vi "ProstSpecFormat.vi"(1 "Spectra.txt old (string)":string) -> (0 "Spectra.txt new out":string)   [LabVIEW 2022 SP3]
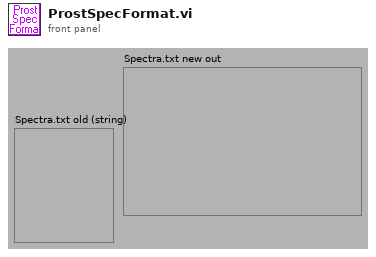
[diagram p1: front panel]
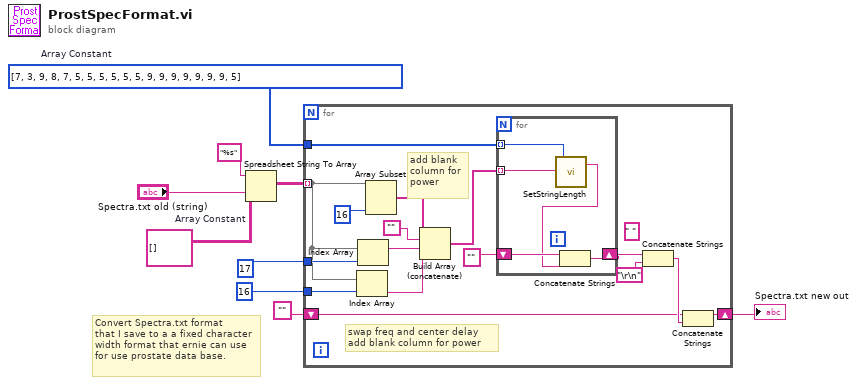
[diagram p0: block diagram]
diagram:
  w6 = i32[] [7, 3, 9, 8, 7, 5, 5, 5, 5, 5, 5, 9, 9, 9, 9, 9, 9, 9, 5]  # Array Constant
  w8 = string[][] []  # Array Constant
  # "Convert Spectra.txt format\nthat I save to a a fixed character\nwidth format that ernie can use\nfor use prostate data base."
  n1 = Spreadsheet String To Array(format string="%s", spreadsheet string="Spectra.txt old (string)", array type (2D Dbl)=w8) -> (array=w7:string[][])  [unwired: 1 out]
  n2 = for {
    tunnel: w7 -> [w10] mode=indexing
    tunnel: w6 -> [w25]
    shift-right: [w23] -> w2
    shift-left: "" -> [w19]
    tunnel: 17 -> [w18]
    tunnel: 16 -> [w17]
    (unwired) " "
    # "add blank\ncolumn for\npower"
    # "swap freq and center delay add blank column for power"
    n3 = Index Array(array=w10, index=w17) -> (element=w14:string)
    n4 = Index Array(array=w10, index=w18) -> (element=w15:string)
    n5 = Array Subset(array=w10, length=16) -> (w13:string[])  [unwired: 1 in]
    n6 = Build Array (concatenate)(w13, "", w15, w14) -> (w11:string[])
    n7 = for {
      tunnel: w25 -> [w30] mode=indexing
      shift-right: [w29] -> w20
      shift-left: "" -> [w28]
      tunnel: w11 -> [w26] mode=indexing
      n8 = call "SetStringLength.vi"("Input String"=w26, "String Length"=w30) -> ("Output String"=w27:string)  [unwired: 1 out]
      n9 = Concatenate Strings(w28, w27) -> (w29:string)
    }
    n10 = Concatenate Strings(w20, "\r\n") -> (w22:string)
    n11 = Concatenate Strings(w19, w22) -> (w23:string)
  }
  "Spectra.txt new out" <- w2
